vi "Instrument.Oxford1820.getAll.vi"(8 "error in (no error)":errorcluster, 11 "Instrument.Oxford1820 in":refnum<class "Instrument.Oxford1820.lvclass">) -> (0 "error out":errorcluster, 2 "output cluster":T1, 3 "Instrument.Oxford1820 out":refnum<class "Instrument.Oxford1820.lvclass">)   [LabVIEW 2019, in "Instrument.Oxford1820.lvclass"]
uses:
  Instrument.Oxford1820.lvclass
  Typedefs/getAll.ctl
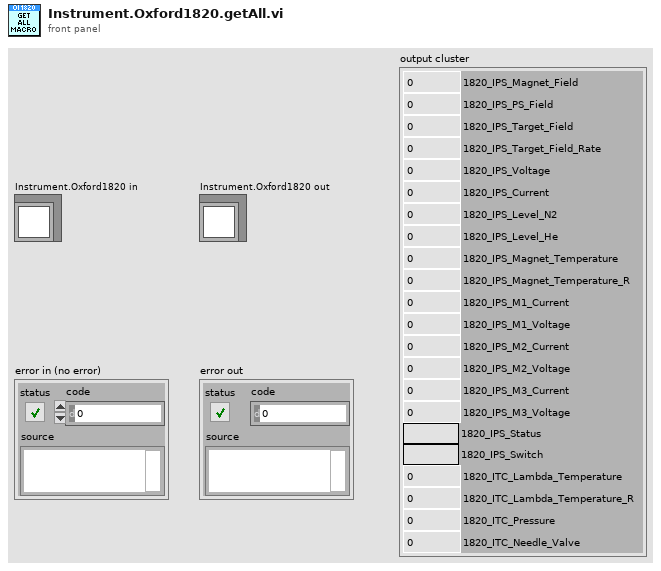
[diagram p1: front panel]
types:
  T1 = typedef "Instrument.Oxford1820.lvclass/getAll.ctl" = cluster{"1820_IPS_Magnet_Field":dbl, "1820_IPS_PS_Field":dbl, "1820_IPS_Target_Field":dbl, "1820_IPS_Target_Field_Rate":dbl, "1820_IPS_Voltage":dbl, "1820_IPS_Current":dbl, "1820_IPS_Level_N2":dbl, "1820_IPS_Level_He":dbl, "1820_IPS_Magnet_Temperature":dbl, "1820_IPS_Magnet_Temperature_R":dbl, "1820_IPS_M1_Current":dbl, "1820_IPS_M1_Voltage":dbl, "1820_IPS_M2_Current":dbl, "1820_IPS_M2_Voltage":dbl, "1820_IPS_M3_Current":dbl, "1820_IPS_M3_Voltage":dbl, "1820_IPS_Status":string, "1820_IPS_Switch":string, "1820_ITC_Lambda_Temperature":dbl, "1820_ITC_Lambda_Temperature_R":dbl, "1820_ITC_Pressure":dbl, "1820_ITC_Needle_Valve":dbl}
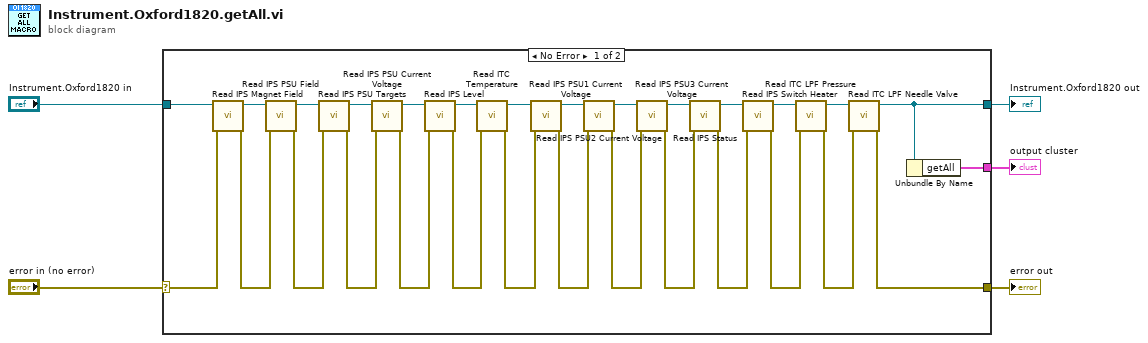
[diagram p0: block diagram]
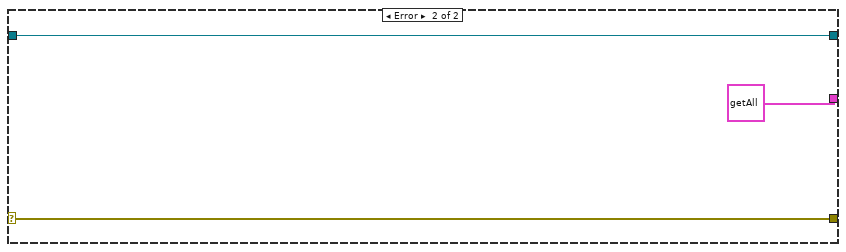
[diagram p2: hidden frame]
diagram:
  n1 = case shown="No Error" "error in (no error)" {
    selector: "error in (no error)" -> [w34 w37]
    tunnel: "Instrument.Oxford1820 in" -> [w7 w36]
    tunnel: [w8 T1 {"1820_IPS_Magnet_Field"=0.0, "1820_IPS_PS_Field"=0.0, "1820_IPS_Target_Field"=0.0, "1820_IPS_Target_Field_Rate"=0.0, "1820_IPS_Voltage"=0.0, "1820_IPS_Current"=0.0, "1820_IPS_Level_N2"=0.0, "1820_IPS_Level_He"=0.0, "1820_IPS_Magnet_Temperature"=0.0, "1820_IPS_Magnet_Temperature_R"=0.0, "1820_IPS_M1_Current"=0.0, "1820_IPS_M1_Voltage"=0.0, "1820_IPS_M2_Current"=0.0, "1820_IPS_M2_Voltage"=0.0, "1820_IPS_M3_Current"=0.0, "1820_IPS_M3_Voltage"=0.0, "1820_IPS_Status"="", "1820_IPS_Switch"="", "1820_ITC_Lambda_Temperature"=0.0, "1820_ITC_Lambda_Temperature_R"=0.0, "1820_ITC_Pressure"=0.0, "1820_ITC_Needle_Valve"=0.0} ("getAll")] -> w3
    tunnel: [w6 w36] -> w2
    tunnel: [w9 w37] -> w1
    frame No Error {
      n2 = call "Read IPS Magnet Field.vi"("error in (no error)"=w34, "Instrument.Oxford1820 in"=w7) -> ("error out"=w11:errorcluster, "Instrument.Oxford1820 out"=w10:refnum<class "Instrument.Oxford1820.lvclass">)  [unwired: 7 in, 1 out]
      n3 = call "Read IPS PSU Field.vi"("error in (no error)"=w11, "Instrument.Oxford1820 in"=w10) -> ("error out"=w13:errorcluster, "Instrument.Oxford1820 out"=w12:refnum<class "Instrument.Oxford1820.lvclass">)  [unwired: 7 in, 1 out]
      n4 = call "Read IPS PSU Targets.vi"("error in (no error)"=w13, "Instrument.Oxford1820 in"=w12) -> ("error out"=w15:errorcluster, "Instrument.Oxford1820 out"=w14:refnum<class "Instrument.Oxford1820.lvclass">)  [unwired: 6 in, 2 out]
      n5 = call "Read IPS PSU Current Voltage.vi"("error in (no error)"=w15, "Instrument.Oxford1820 in"=w14) -> ("error out"=w17:errorcluster, "Instrument.Oxford1820 out"=w16:refnum<class "Instrument.Oxford1820.lvclass">)  [unwired: 6 in, 2 out]
      n6 = call "Read IPS Level.vi"("error in (no error)"=w17, "Instrument.Oxford1820 in"=w16) -> ("error out"=w31:errorcluster, "Instrument.Oxford1820 out"=w30:refnum<class "Instrument.Oxford1820.lvclass">)  [unwired: 6 in, 2 out]
      n7 = call "Read ITC Temperature.vi"("error in (no error)"=w31, "Instrument.Oxford1820 in"=w30) -> ("error out"=w32:errorcluster, "Instrument.Oxford1820 out"=w33:refnum<class "Instrument.Oxford1820.lvclass">)  [unwired: 6 in, 2 out]
      n8 = call "Read IPS PSU1 Current Voltage.vi"("error in (no error)"=w32, "Instrument.Oxford1820 in"=w33) -> ("error out"=w19:errorcluster, "Instrument.Oxford1820 out"=w18:refnum<class "Instrument.Oxford1820.lvclass">)  [unwired: 6 in, 2 out]
      n9 = call "Read IPS PSU2 Current Voltage.vi"("error in (no error)"=w19, "Instrument.Oxford1820 in"=w18) -> ("error out"=w21:errorcluster, "Instrument.Oxford1820 out"=w20:refnum<class "Instrument.Oxford1820.lvclass">)  [unwired: 6 in, 2 out]
      n10 = call "Read IPS PSU3 Current Voltage.vi"("error in (no error)"=w21, "Instrument.Oxford1820 in"=w20) -> ("error out"=w23:errorcluster, "Instrument.Oxford1820 out"=w22:refnum<class "Instrument.Oxford1820.lvclass">)  [unwired: 6 in, 2 out]
      n11 = call "Read IPS Status.vi"("error in (no error)"=w23, "Instrument.Oxford1820 in"=w22) -> ("error out"=w25:errorcluster, "Instrument.Oxford1820 out"=w24:refnum<class "Instrument.Oxford1820.lvclass">)  [unwired: 7 in, 1 out]
      n12 = call "Read IPS Switch Heater.vi"("error in (no error)"=w25, "Instrument.Oxford1820 in"=w24) -> ("error out"=w27:errorcluster, "Instrument.Oxford1820 out"=w26:refnum<class "Instrument.Oxford1820.lvclass">)  [unwired: 6 in, 2 out]
      n13 = call "Read ITC LPF Pressure.vi"("error in (no error)"=w27, "Instrument.Oxford1820 in"=w26) -> ("error out"=w29:errorcluster, "Instrument.Oxford1820 out"=w28:refnum<class "Instrument.Oxford1820.lvclass">)  [unwired: 7 in, 1 out]
      n14 = call "Read ITC LPF Needle Valve.vi"("error in (no error)"=w29, "Instrument.Oxford1820 in"=w28) -> ("error out"=w9:errorcluster, "Instrument.Oxford1820 out"=w6:refnum<class "Instrument.Oxford1820.lvclass">)  [unwired: 7 in, 1 out]
      n15 = Unbundle By Name(w6) -> ("getAll"=w8:T1)
    }
    frame Error {
    }
  }
  "output cluster" <- w3
  "Instrument.Oxford1820 out" <- w2
  "error out" <- w1
